vi "Text_help.vi"(6 "Onto":bool[](array[boolean]), 7 "Trigger Array":bool[](array[boolean]), 9 "Changed":bool, 10 "Bounds":T2[](array[typedef]), 11 "Refs cluster In":T1) -> (3 "Refs cluster Out":T1)   [LabVIEW 2015]
uses:
  <vilib>/Utility/miscctls.llb/LVRectTypeDef.ctl
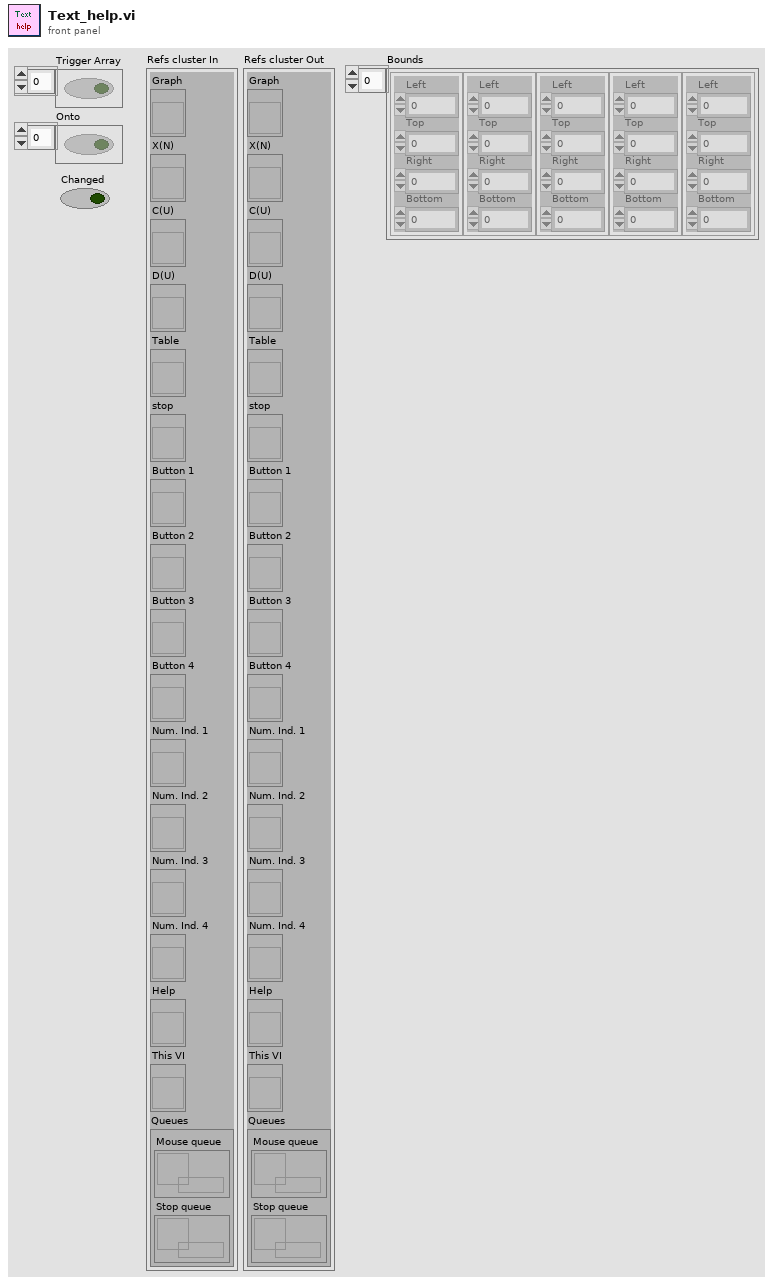
[diagram p1: front panel]
types:
  T1 = cluster{"Graph":refnum<vi>, "X(N)":refnum<vi>, "C(U)":refnum<vi>, "D(U)":refnum<vi>, "Table":refnum<vi>, "stop":refnum<vi>, "Button 1":refnum<vi>, "Button 2":refnum<vi>, "Button 3":refnum<vi>, "Button 4":refnum<vi>, "Num. Ind. 1":refnum<vi>, "Num. Ind. 2":refnum<vi>, "Num. Ind. 3":refnum<vi>, "Num. Ind. 4":refnum<vi>, "Help":refnum<vi>, "This VI":refnum<vi>, "Queues":cluster{"Mouse queue":refnum<queue>, "Stop queue":refnum<queue>}}
  T2 = typedef "LVRectTypeDef.ctl" = cluster{"Left":i16, "Top":i16, "Right":i16, "Bottom":i16}
  T3 = enum16{"top-left", "top-right", "bot-left", "bot-right"}
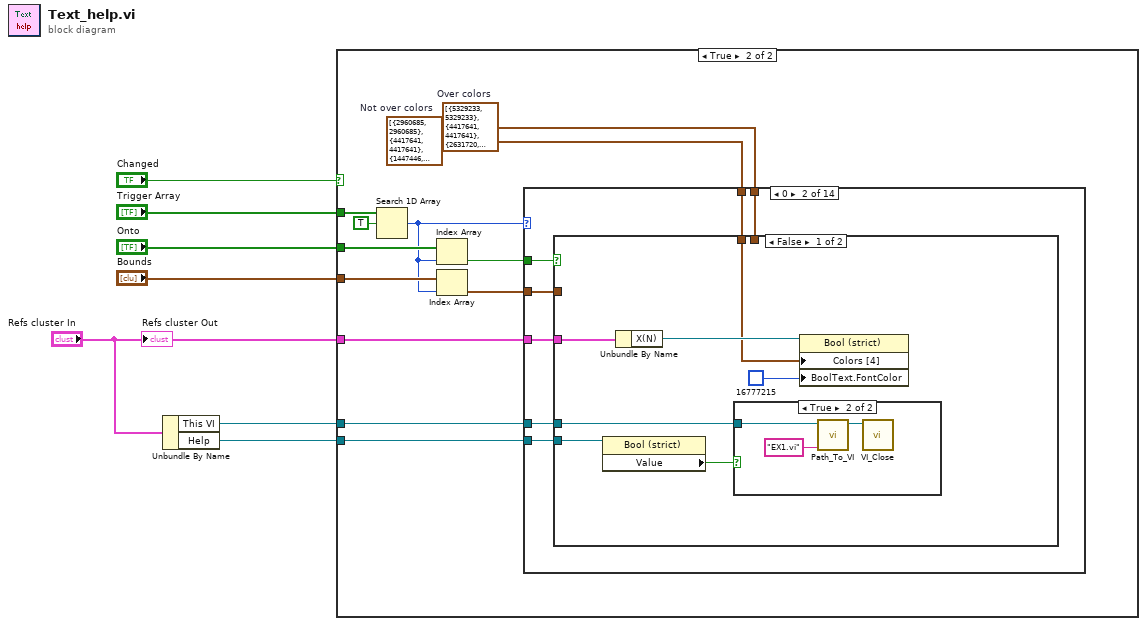
[diagram p0: block diagram]
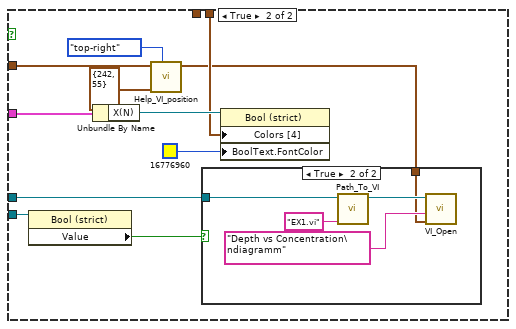
[diagram p5: hidden frame]
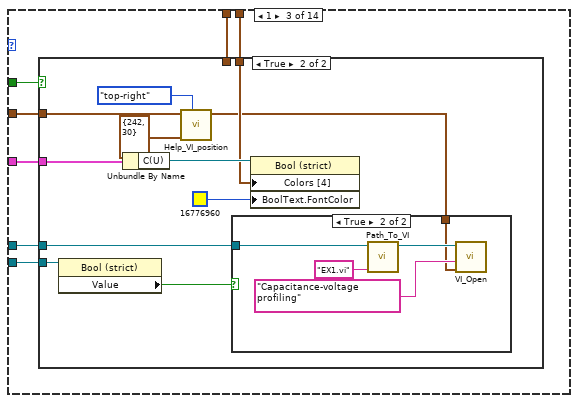
[diagram p7: hidden frame]
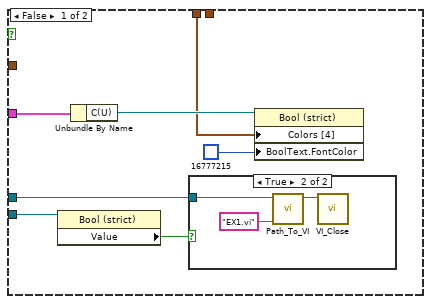
[diagram p8: hidden frame]
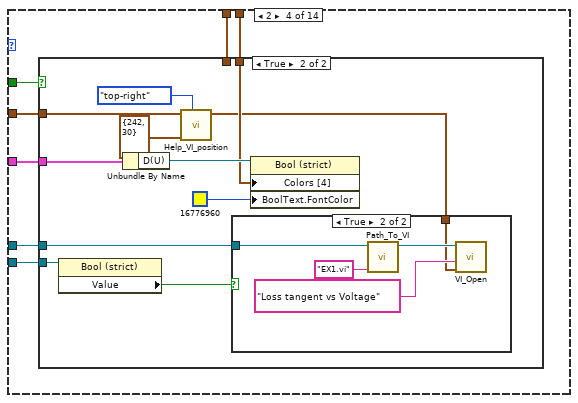
[diagram p11: hidden frame]
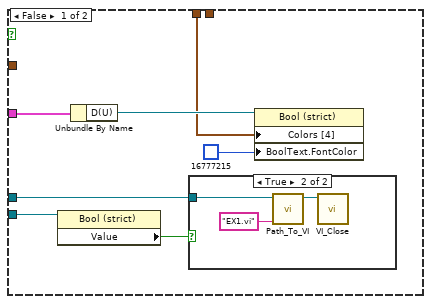
[diagram p12: hidden frame]
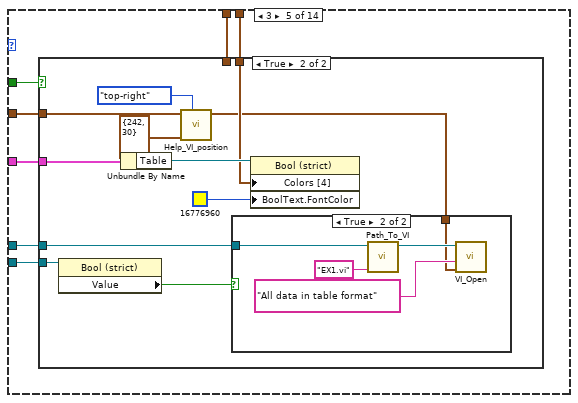
[diagram p15: hidden frame]
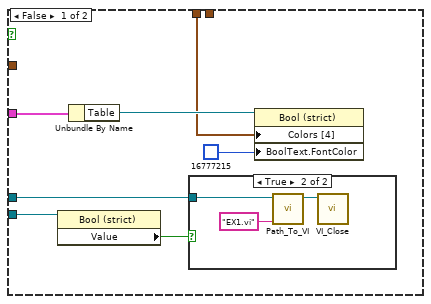
[diagram p16: hidden frame]
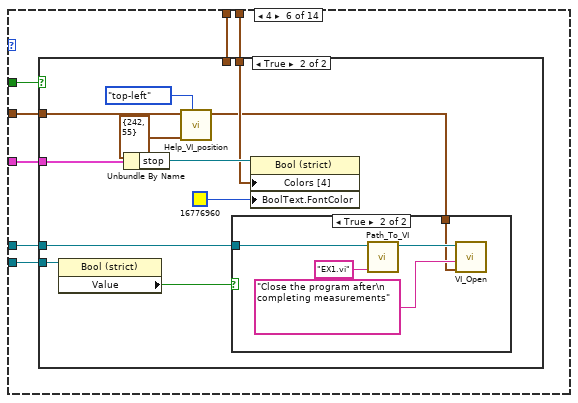
[diagram p19: hidden frame]
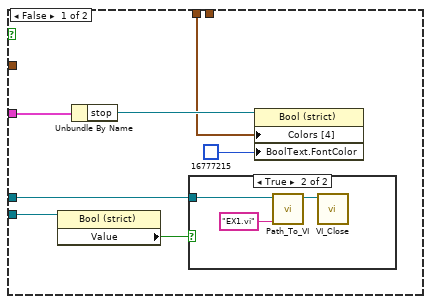
[diagram p20: hidden frame]
diagram:
  n1 = Unbundle By Name("Refs cluster In") -> ("This VI"=w2:refnum<vi>, "Help"=w1:refnum<vi>)
  n2 = case shown="True" "Changed" {
    tunnel: "Refs cluster In" -> [_ w15]
    tunnel: "Trigger Array" -> [_ w19]
    tunnel: "Onto" -> [_ w17]
    tunnel: "Bounds" -> [_ w14]
    tunnel: w2 -> [_ w9]
    tunnel: w1 -> [_ w8]
    frame False {
    }
    frame True {
      w10 = cluster{u32, u32}[] [{2960685, 2960685}, {4417641, 4417641}, {1447446, 1447446}, {2176052, 2176052}]  # Not over colors
      w11 = cluster{u32, u32}[] [{5329233, 5329233}, {4417641, 4417641}, {2631720, 2631720}, {2176052, 2176052}]  # Over colors
      n3 = Search 1D Array(1D array=w19, element=TRUE) -> (index of element=w13:i32)  [unwired: 1 in]
      n4 = Index Array(array=w17, index=w13) -> (element=w16:bool)
      n5 = Index Array(array=w14, index=w13) -> (element=w12:T2)
      n6 = case shown="0" w13 {
        tunnel: w16 -> [_ w25 w58 w91 w124 w157 w190 w223 w256 w289 w322 w355 w388 w421]
        tunnel: w15 -> [_ w26 w59 w92 w125 w158 w191 w224 w257 w290 w323 w356 w389 w422]
        tunnel: w12 -> [_ w24 w57 w90 w123 w156 w189 w222 w255 w288 w321 w354 w387 w420]
        tunnel: w11 -> [_ w22 w55 w88 w121 w154 w187 w220 w253 w286 w319 w352 w385 w418]
        tunnel: w10 -> [_ w21 w54 w87 w120 w153 w186 w219 w252 w285 w318 w351 w384 w417]
        tunnel: w9 -> [_ w23 w56 w89 w122 w155 w188 w221 w254 w287 w320 w353 w386 w419]
        tunnel: w8 -> [_ w20 w53 w86 w119 w152 w185 w218 w251 w284 w317 w350 w383 w416]
        frame -1, Default {
        }
        frame 0 {
          n7 = case shown="False" w25 {
            tunnel: w26 -> [w33 w47]
            tunnel: w24 -> [_ w40]
            tunnel: w23 -> [w29 w46]
            tunnel: w22 -> [_ w43]
            tunnel: w21 -> [w30 _]
            tunnel: w20 -> [w28 w38]
            frame False {
              n8 = property class="Bool (strict)"(reference=w28) -> ("Value"=w27:bool)  [unwired: 1 in, 2 out]
              n9 = Unbundle By Name(w33) -> ("X(N)"=w32:refnum<vi>)
              n10 = case shown="True" w27 {
                tunnel: w29 -> [_ w34]
                frame False {
                }
                frame True {
                  n11 = call "Path_To_VI.vi"("Vi name (with .vi)"="EX1.vi", "This Vi ref"=w34) -> ("Opening VI reference"=w36:refnum<vi>)  [unwired: 9 in]
                  n12 = call "VI_Close.vi"("VI_In"=w36) -> ()  [unwired: 10 in, 1 out]
                }
              }
              n13 = property on="Property Node" class="Bool (strict)"(reference=w32, "Colors [4]"=w30, "BoolText.FontColor"=u32 16777215) -> ()  [unwired: 1 in, 2 out]
            }
            frame True {
              n14 = property class="Bool (strict)"(reference=w38) -> ("Value"=w37:bool)  [unwired: 1 in, 2 out]
              n15 = Unbundle By Name(w47) -> ("X(N)"=w45:refnum<vi>)
              n16 = call "Help_VI_position.vi"("Enum"=T3."top-right", "Width-Height"=cluster{"width":i16, "height":i16} {"width"=242, "height"=55}, "Bounds button"=w40) -> ("Panel Bounds"=w39:T2)  [unwired: 8 in]
              n17 = case shown="True" w37 {
                tunnel: w46 -> [_ w49]
                tunnel: w39 -> [_ w48]
                frame False {
                }
                frame True {
                  n18 = call "Path_To_VI.vi"("Vi name (with .vi)"="EX1.vi", "This Vi ref"=w49) -> ("Opening VI reference"=w50:refnum<vi>)  [unwired: 9 in]
                  n19 = call "VI_Open.vi"("Panel Bounds"=w48, "Строка help"="Depth vs Concentration\ndiagramm", "Current VI In"=w50) -> ()  [unwired: 8 in, 1 out]
                }
              }
              n20 = property on="Property Node" class="Bool (strict)"(reference=w45, "Colors [4]"=w43, "BoolText.FontColor"=u32 16776960) -> ()  [unwired: 1 in, 2 out]
            }
          }
        }
        frame 1 {
          n21 = case shown="True" w58 {
            tunnel: w59 -> [w66 w80]
            tunnel: w57 -> [_ w73]
            tunnel: w56 -> [w62 w79]
            tunnel: w55 -> [_ w76]
            tunnel: w54 -> [w63 _]
            tunnel: w53 -> [w61 w71]
            frame False {
              n22 = property class="Bool (strict)"(reference=w61) -> ("Value"=w60:bool)  [unwired: 1 in, 2 out]
              n23 = Unbundle By Name(w66) -> ("C(U)"=w65:refnum<vi>)
              n24 = case shown="True" w60 {
                tunnel: w62 -> [_ w67]
                frame False {
                }
                frame True {
                  n25 = call "Path_To_VI.vi"("Vi name (with .vi)"="EX1.vi", "This Vi ref"=w67) -> ("Opening VI reference"=w69:refnum<vi>)  [unwired: 9 in]
                  n26 = call "VI_Close.vi"("VI_In"=w69) -> ()  [unwired: 10 in, 1 out]
                }
              }
              n27 = property on="Property Node" class="Bool (strict)"(reference=w65, "Colors [4]"=w63, "BoolText.FontColor"=u32 16777215) -> ()  [unwired: 1 in, 2 out]
            }
            frame True {
              n28 = property class="Bool (strict)"(reference=w71) -> ("Value"=w70:bool)  [unwired: 1 in, 2 out]
              n29 = Unbundle By Name(w80) -> ("C(U)"=w78:refnum<vi>)
              n30 = call "Help_VI_position.vi"("Enum"=T3."top-right", "Width-Height"=cluster{"width":i16, "height":i16} {"width"=242, "height"=30}, "Bounds button"=w73) -> ("Panel Bounds"=w72:T2)  [unwired: 8 in]
              n31 = case shown="True" w70 {
                tunnel: w79 -> [_ w82]
                tunnel: w72 -> [_ w81]
                frame False {
                }
                frame True {
                  n32 = call "Path_To_VI.vi"("Vi name (with .vi)"="EX1.vi", "This Vi ref"=w82) -> ("Opening VI reference"=w83:refnum<vi>)  [unwired: 9 in]
                  n33 = call "VI_Open.vi"("Panel Bounds"=w81, "Строка help"="Capacitance-voltage profiling", "Current VI In"=w83) -> ()  [unwired: 8 in, 1 out]
                }
              }
              n34 = property on="Property Node" class="Bool (strict)"(reference=w78, "Colors [4]"=w76, "BoolText.FontColor"=u32 16776960) -> ()  [unwired: 1 in, 2 out]
            }
          }
        }
        frame 2 {
          n35 = case shown="True" w91 {
            tunnel: w92 -> [w99 w113]
            tunnel: w90 -> [_ w106]
            tunnel: w89 -> [w95 w112]
            tunnel: w88 -> [_ w109]
            tunnel: w87 -> [w96 _]
            tunnel: w86 -> [w94 w104]
            frame False {
              n36 = property class="Bool (strict)"(reference=w94) -> ("Value"=w93:bool)  [unwired: 1 in, 2 out]
              n37 = Unbundle By Name(w99) -> ("D(U)"=w98:refnum<vi>)
              n38 = case shown="True" w93 {
                tunnel: w95 -> [_ w100]
                frame False {
                }
                frame True {
                  n39 = call "Path_To_VI.vi"("Vi name (with .vi)"="EX1.vi", "This Vi ref"=w100) -> ("Opening VI reference"=w102:refnum<vi>)  [unwired: 9 in]
                  n40 = call "VI_Close.vi"("VI_In"=w102) -> ()  [unwired: 10 in, 1 out]
                }
              }
              n41 = property on="Property Node" class="Bool (strict)"(reference=w98, "Colors [4]"=w96, "BoolText.FontColor"=u32 16777215) -> ()  [unwired: 1 in, 2 out]
            }
            frame True {
              n42 = property class="Bool (strict)"(reference=w104) -> ("Value"=w103:bool)  [unwired: 1 in, 2 out]
              n43 = Unbundle By Name(w113) -> ("D(U)"=w111:refnum<vi>)
              n44 = call "Help_VI_position.vi"("Enum"=T3."top-right", "Width-Height"=cluster{"width":i16, "height":i16} {"width"=242, "height"=30}, "Bounds button"=w106) -> ("Panel Bounds"=w105:T2)  [unwired: 8 in]
              n45 = case shown="True" w103 {
                tunnel: w112 -> [_ w115]
                tunnel: w105 -> [_ w114]
                frame False {
                }
                frame True {
                  n46 = call "Path_To_VI.vi"("Vi name (with .vi)"="EX1.vi", "This Vi ref"=w115) -> ("Opening VI reference"=w116:refnum<vi>)  [unwired: 9 in]
                  n47 = call "VI_Open.vi"("Panel Bounds"=w114, "Строка help"="Loss tangent vs Voltage", "Current VI In"=w116) -> ()  [unwired: 8 in, 1 out]
                }
              }
              n48 = property on="Property Node" class="Bool (strict)"(reference=w111, "Colors [4]"=w109, "BoolText.FontColor"=u32 16776960) -> ()  [unwired: 1 in, 2 out]
            }
          }
        }
        frame 3 {
          n49 = case shown="True" w124 {
            tunnel: w125 -> [w132 w146]
            tunnel: w123 -> [_ w139]
            tunnel: w122 -> [w128 w145]
            tunnel: w121 -> [_ w142]
            tunnel: w120 -> [w129 _]
            tunnel: w119 -> [w127 w137]
            frame False {
              n50 = property class="Bool (strict)"(reference=w127) -> ("Value"=w126:bool)  [unwired: 1 in, 2 out]
              n51 = Unbundle By Name(w132) -> ("Table"=w131:refnum<vi>)
              n52 = case shown="True" w126 {
                tunnel: w128 -> [_ w133]
                frame False {
                }
                frame True {
                  n53 = call "Path_To_VI.vi"("Vi name (with .vi)"="EX1.vi", "This Vi ref"=w133) -> ("Opening VI reference"=w135:refnum<vi>)  [unwired: 9 in]
                  n54 = call "VI_Close.vi"("VI_In"=w135) -> ()  [unwired: 10 in, 1 out]
                }
              }
              n55 = property on="Property Node" class="Bool (strict)"(reference=w131, "Colors [4]"=w129, "BoolText.FontColor"=u32 16777215) -> ()  [unwired: 1 in, 2 out]
            }
            frame True {
              n56 = property class="Bool (strict)"(reference=w137) -> ("Value"=w136:bool)  [unwired: 1 in, 2 out]
              n57 = Unbundle By Name(w146) -> ("Table"=w144:refnum<vi>)
              n58 = call "Help_VI_position.vi"("Enum"=T3."top-right", "Width-Height"=cluster{"width":i16, "height":i16} {"width"=242, "height"=30}, "Bounds button"=w139) -> ("Panel Bounds"=w138:T2)  [unwired: 8 in]
              n59 = case shown="True" w136 {
                tunnel: w145 -> [_ w148]
                tunnel: w138 -> [_ w147]
                frame False {
                }
                frame True {
                  n60 = call "Path_To_VI.vi"("Vi name (with .vi)"="EX1.vi", "This Vi ref"=w148) -> ("Opening VI reference"=w149:refnum<vi>)  [unwired: 9 in]
                  n61 = call "VI_Open.vi"("Panel Bounds"=w147, "Строка help"="All data in table format", "Current VI In"=w149) -> ()  [unwired: 8 in, 1 out]
                }
              }
              n62 = property on="Property Node" class="Bool (strict)"(reference=w144, "Colors [4]"=w142, "BoolText.FontColor"=u32 16776960) -> ()  [unwired: 1 in, 2 out]
            }
          }
        }
        frame 4 {
          n63 = case shown="True" w157 {
            tunnel: w158 -> [w165 w179]
            tunnel: w156 -> [_ w172]
            tunnel: w155 -> [w161 w178]
            tunnel: w154 -> [_ w175]
            tunnel: w153 -> [w162 _]
            tunnel: w152 -> [w160 w170]
            frame False {
              n64 = property class="Bool (strict)"(reference=w160) -> ("Value"=w159:bool)  [unwired: 1 in, 2 out]
              n65 = Unbundle By Name(w165) -> ("stop"=w164:refnum<vi>)
              n66 = case shown="True" w159 {
                tunnel: w161 -> [_ w166]
                frame False {
                }
                frame True {
                  n67 = call "Path_To_VI.vi"("Vi name (with .vi)"="EX1.vi", "This Vi ref"=w166) -> ("Opening VI reference"=w168:refnum<vi>)  [unwired: 9 in]
                  n68 = call "VI_Close.vi"("VI_In"=w168) -> ()  [unwired: 10 in, 1 out]
                }
              }
              n69 = property on="Property Node" class="Bool (strict)"(reference=w164, "Colors [4]"=w162, "BoolText.FontColor"=u32 16777215) -> ()  [unwired: 1 in, 2 out]
            }
            frame True {
              n70 = property class="Bool (strict)"(reference=w170) -> ("Value"=w169:bool)  [unwired: 1 in, 2 out]
              n71 = Unbundle By Name(w179) -> ("stop"=w177:refnum<vi>)
              n72 = call "Help_VI_position.vi"("Enum"=T3."top-left", "Width-Height"=cluster{"width":i16, "height":i16} {"width"=242, "height"=55}, "Bounds button"=w172) -> ("Panel Bounds"=w171:T2)  [unwired: 8 in]
              n73 = case shown="True" w169 {
                tunnel: w178 -> [_ w181]
                tunnel: w171 -> [_ w180]
                frame False {
                }
                frame True {
                  n74 = call "Path_To_VI.vi"("Vi name (with .vi)"="EX1.vi", "This Vi ref"=w181) -> ("Opening VI reference"=w182:refnum<vi>)  [unwired: 9 in]
                  n75 = call "VI_Open.vi"("Panel Bounds"=w180, "Строка help"="Close the program after\n completing measurements", "Current VI In"=w182) -> ()  [unwired: 8 in, 1 out]
                }
              }
              n76 = property on="Property Node" class="Bool (strict)"(reference=w177, "Colors [4]"=w175, "BoolText.FontColor"=u32 16776960) -> ()  [unwired: 1 in, 2 out]
            }
          }
        }
        frame 5 {
          n77 = case shown="True" w190 {
            tunnel: w191 -> [w198 w212]
            tunnel: w189 -> [_ w205]
            tunnel: w188 -> [w194 w211]
            tunnel: w187 -> [_ w208]
            tunnel: w186 -> [w195 _]
            tunnel: w185 -> [w193 w203]
            frame False {
              n78 = property class="Bool (strict)"(reference=w193) -> ("Value"=w192:bool)  [unwired: 1 in, 2 out]
              n79 = Unbundle By Name(w198) -> ("Button 1"=w197:refnum<vi>)
              n80 = case shown="True" w192 {
                tunnel: w194 -> [_ w199]
                frame False {
                }
                frame True {
                  n81 = call "Path_To_VI.vi"("Vi name (with .vi)"="EX1.vi", "This Vi ref"=w199) -> ("Opening VI reference"=w201:refnum<vi>)  [unwired: 9 in]
                  n82 = call "VI_Close.vi"("VI_In"=w201) -> ()  [unwired: 10 in, 1 out]
                }
              }
              n83 = property on="Property Node" class="Bool (strict)"(reference=w197, "Colors [4]"=w195, "BoolText.FontColor"=u32 16777215) -> ()  [unwired: 1 in, 2 out]
            }
            frame True {
              n84 = property class="Bool (strict)"(reference=w203) -> ("Value"=w202:bool)  [unwired: 1 in, 2 out]
              n85 = Unbundle By Name(w212) -> ("Button 1"=w210:refnum<vi>)
              n86 = call "Help_VI_position.vi"("Enum"=T3."bot-left", "Width-Height"=cluster{"width":i16, "height":i16} {"width"=242, "height"=30}, "Bounds button"=w205) -> ("Panel Bounds"=w204:T2)  [unwired: 8 in]
              n87 = case shown="True" w202 {
                tunnel: w211 -> [_ w214]
                tunnel: w204 -> [_ w213]
                frame False {
                }
                frame True {
                  n88 = call "Path_To_VI.vi"("Vi name (with .vi)"="EX1.vi", "This Vi ref"=w214) -> ("Opening VI reference"=w215:refnum<vi>)  [unwired: 9 in]
                  n89 = call "VI_Open.vi"("Panel Bounds"=w213, "Строка help"="Text for button #1", "Current VI In"=w215) -> ()  [unwired: 8 in, 1 out]
                }
              }
              n90 = property on="Property Node" class="Bool (strict)"(reference=w210, "Colors [4]"=w208, "BoolText.FontColor"=u32 16776960) -> ()  [unwired: 1 in, 2 out]
            }
          }
        }
        frame 6 {
          n91 = case shown="True" w223 {
            tunnel: w224 -> [w231 w245]
            tunnel: w222 -> [_ w238]
            tunnel: w221 -> [w227 w244]
            tunnel: w220 -> [_ w241]
            tunnel: w219 -> [w228 _]
            tunnel: w218 -> [w226 w236]
            frame False {
              n92 = property class="Bool (strict)"(reference=w226) -> ("Value"=w225:bool)  [unwired: 1 in, 2 out]
              n93 = Unbundle By Name(w231) -> ("Button 2"=w230:refnum<vi>)
              n94 = case shown="True" w225 {
                tunnel: w227 -> [_ w232]
                frame False {
                }
                frame True {
                  n95 = call "Path_To_VI.vi"("Vi name (with .vi)"="EX1.vi", "This Vi ref"=w232) -> ("Opening VI reference"=w234:refnum<vi>)  [unwired: 9 in]
                  n96 = call "VI_Close.vi"("VI_In"=w234) -> ()  [unwired: 10 in, 1 out]
                }
              }
              n97 = property on="Property Node" class="Bool (strict)"(reference=w230, "Colors [4]"=w228, "BoolText.FontColor"=u32 16777215) -> ()  [unwired: 1 in, 2 out]
            }
            frame True {
              n98 = property class="Bool (strict)"(reference=w236) -> ("Value"=w235:bool)  [unwired: 1 in, 2 out]
              n99 = Unbundle By Name(w245) -> ("Button 2"=w243:refnum<vi>)
              n100 = call "Help_VI_position.vi"("Enum"=T3."top-left", "Width-Height"=cluster{"width":i16, "height":i16} {"width"=242, "height"=30}, "Bounds button"=w238) -> ("Panel Bounds"=w237:T2)  [unwired: 8 in]
              n101 = case shown="True" w235 {
                tunnel: w244 -> [_ w247]
                tunnel: w237 -> [_ w246]
                frame False {
                }
                frame True {
                  n102 = call "Path_To_VI.vi"("Vi name (with .vi)"="EX1.vi", "This Vi ref"=w247) -> ("Opening VI reference"=w248:refnum<vi>)  [unwired: 9 in]
                  n103 = call "VI_Open.vi"("Panel Bounds"=w246, "Строка help"="Text for button #2", "Current VI In"=w248) -> ()  [unwired: 8 in, 1 out]
                }
              }
              n104 = property on="Property Node" class="Bool (strict)"(reference=w243, "Colors [4]"=w241, "BoolText.FontColor"=u32 16776960) -> ()  [unwired: 1 in, 2 out]
            }
          }
        }
        frame 7 {
          n105 = case shown="True" w256 {
            tunnel: w257 -> [w264 w278]
            tunnel: w255 -> [_ w271]
            tunnel: w254 -> [w260 w277]
            tunnel: w253 -> [_ w274]
            tunnel: w252 -> [w261 _]
            tunnel: w251 -> [w259 w269]
            frame False {
              n106 = property class="Bool (strict)"(reference=w259) -> ("Value"=w258:bool)  [unwired: 1 in, 2 out]
              n107 = Unbundle By Name(w264) -> ("Button 3"=w263:refnum<vi>)
              n108 = case shown="True" w258 {
                tunnel: w260 -> [_ w265]
                frame False {
                }
                frame True {
                  n109 = call "Path_To_VI.vi"("Vi name (with .vi)"="EX1.vi", "This Vi ref"=w265) -> ("Opening VI reference"=w267:refnum<vi>)  [unwired: 9 in]
                  n110 = call "VI_Close.vi"("VI_In"=w267) -> ()  [unwired: 10 in, 1 out]
                }
              }
              n111 = property on="Property Node" class="Bool (strict)"(reference=w263, "Colors [4]"=w261, "BoolText.FontColor"=u32 16777215) -> ()  [unwired: 1 in, 2 out]
            }
            frame True {
              n112 = property class="Bool (strict)"(reference=w269) -> ("Value"=w268:bool)  [unwired: 1 in, 2 out]
              n113 = Unbundle By Name(w278) -> ("Button 3"=w276:refnum<vi>)
              n114 = call "Help_VI_position.vi"("Enum"=T3."top-left", "Width-Height"=cluster{"width":i16, "height":i16} {"width"=242, "height"=30}, "Bounds button"=w271) -> ("Panel Bounds"=w270:T2)  [unwired: 8 in]
              n115 = case shown="True" w268 {
                tunnel: w277 -> [_ w280]
                tunnel: w270 -> [_ w279]
                frame False {
                }
                frame True {
                  n116 = call "Path_To_VI.vi"("Vi name (with .vi)"="EX1.vi", "This Vi ref"=w280) -> ("Opening VI reference"=w281:refnum<vi>)  [unwired: 9 in]
                  n117 = call "VI_Open.vi"("Panel Bounds"=w279, "Строка help"="Text for button #3", "Current VI In"=w281) -> ()  [unwired: 8 in, 1 out]
                }
              }
              n118 = property on="Property Node" class="Bool (strict)"(reference=w276, "Colors [4]"=w274, "BoolText.FontColor"=u32 16776960) -> ()  [unwired: 1 in, 2 out]
            }
          }
        }
        frame 8 {
          n119 = case shown="True" w289 {
            tunnel: w290 -> [w297 w311]
            tunnel: w288 -> [_ w304]
            tunnel: w287 -> [w293 w310]
            tunnel: w286 -> [_ w307]
            tunnel: w285 -> [w294 _]
            tunnel: w284 -> [w292 w302]
            frame False {
              n120 = property class="Bool (strict)"(reference=w292) -> ("Value"=w291:bool)  [unwired: 1 in, 2 out]
              n121 = Unbundle By Name(w297) -> ("Button 4"=w296:refnum<vi>)
              n122 = case shown="True" w291 {
                tunnel: w293 -> [_ w298]
                frame False {
                }
                frame True {
                  n123 = call "Path_To_VI.vi"("Vi name (with .vi)"="EX1.vi", "This Vi ref"=w298) -> ("Opening VI reference"=w300:refnum<vi>)  [unwired: 9 in]
                  n124 = call "VI_Close.vi"("VI_In"=w300) -> ()  [unwired: 10 in, 1 out]
                }
              }
              n125 = property on="Property Node" class="Bool (strict)"(reference=w296, "Colors [4]"=w294, "BoolText.FontColor"=u32 16777215) -> ()  [unwired: 1 in, 2 out]
            }
            frame True {
              n126 = property class="Bool (strict)"(reference=w302) -> ("Value"=w301:bool)  [unwired: 1 in, 2 out]
              n127 = Unbundle By Name(w311) -> ("Button 4"=w309:refnum<vi>)
              n128 = call "Help_VI_position.vi"("Enum"=T3."top-left", "Width-Height"=cluster{"width":i16, "height":i16} {"width"=242, "height"=30}, "Bounds button"=w304) -> ("Panel Bounds"=w303:T2)  [unwired: 8 in]
              n129 = case shown="True" w301 {
                tunnel: w310 -> [_ w313]
                tunnel: w303 -> [_ w312]
                frame False {
                }
                frame True {
                  n130 = call "Path_To_VI.vi"("Vi name (with .vi)"="EX1.vi", "This Vi ref"=w313) -> ("Opening VI reference"=w314:refnum<vi>)  [unwired: 9 in]
                  n131 = call "VI_Open.vi"("Panel Bounds"=w312, "Строка help"="Text for button #4", "Current VI In"=w314) -> ()  [unwired: 8 in, 1 out]
                }
              }
              n132 = property on="Property Node" class="Bool (strict)"(reference=w309, "Colors [4]"=w307, "BoolText.FontColor"=u32 16776960) -> ()  [unwired: 1 in, 2 out]
            }
          }
        }
        frame 9 {
          n133 = case shown="True" w322 {
            tunnel: w323 -> [w330 w344]
            tunnel: w321 -> [_ w340]
            tunnel: w320 -> [w329 w343]
            tunnel: w319 -> [_ _]
            tunnel: w318 -> [_ _]
            tunnel: w317 -> [w328 w338]
            frame False {
              n134 = Unbundle By Name(w330) -> ("Num. Ind. 1"=w324:refnum<vi>)
              n135 = property class="Bool (strict)"(reference=w328) -> ("Value"=w327:bool)  [unwired: 1 in, 2 out]
              n136 = property on="Property Node" class="DigNum (strict)"(reference=w324, "NumText.TextColors"=cluster{u32, u32} {16777215, 3815994} ("Cluster"), "Label.TextColor"=u32 16777215) -> ()  [unwired: 1 in, 2 out]
              n137 = case shown="True" w327 {
                tunnel: w329 -> [_ w331]
                frame False {
                }
                frame True {
                  n138 = call "Path_To_VI.vi"("Vi name (with .vi)"="EX1.vi", "This Vi ref"=w331) -> ("Opening VI reference"=w333:refnum<vi>)  [unwired: 9 in]
                  n139 = call "VI_Close.vi"("VI_In"=w333) -> ()  [unwired: 10 in, 1 out]
                }
              }
            }
            frame True {
              n140 = property class="Bool (strict)"(reference=w338) -> ("Value"=w337:bool)  [unwired: 1 in, 2 out]
              n141 = Unbundle By Name(w344) -> ("Num. Ind. 1"=w335:refnum<vi>)
              n142 = call "Help_VI_position.vi"("Enum"=T3."bot-left", "Width-Height"=cluster{"width":i16, "height":i16} {"width"=242, "height"=30}, "Bounds button"=w340) -> ("Panel Bounds"=w339:T2)  [unwired: 8 in]
              n143 = case shown="True" w337 {
                tunnel: w343 -> [_ w346]
                tunnel: w339 -> [_ w345]
                frame False {
                }
                frame True {
                  n144 = call "Path_To_VI.vi"("Vi name (with .vi)"="EX1.vi", "This Vi ref"=w346) -> ("Opening VI reference"=w347:refnum<vi>)  [unwired: 9 in]
                  n145 = call "VI_Open.vi"("Panel Bounds"=w345, "Строка help"="Text for Numeric Indicator #1", "Current VI In"=w347) -> ()  [unwired: 8 in, 1 out]
                }
              }
              n146 = property on="Property Node" class="DigNum (strict)"(reference=w335, "NumText.TextColors"=cluster{u32, u32} {16645629, 5263440}, "Label.TextColor"=u32 16776960) -> ()  [unwired: 1 in, 2 out]
            }
          }
        }
        frame 10 {
          n147 = case shown="True" w355 {
            tunnel: w356 -> [w363 w377]
            tunnel: w354 -> [_ w373]
            tunnel: w353 -> [w362 w376]
            tunnel: w352 -> [_ _]
            tunnel: w351 -> [_ _]
            tunnel: w350 -> [w361 w371]
            frame False {
              n148 = Unbundle By Name(w363) -> ("Num. Ind. 2"=w357:refnum<vi>)
              n149 = property class="Bool (strict)"(reference=w361) -> ("Value"=w360:bool)  [unwired: 1 in, 2 out]
              n150 = property on="Property Node" class="DigNum (strict)"(reference=w357, "NumText.TextColors"=cluster{u32, u32} {16777215, 3815994} ("Cluster"), "Label.TextColor"=u32 16777215) -> ()  [unwired: 1 in, 2 out]
              n151 = case shown="True" w360 {
                tunnel: w362 -> [_ w364]
                frame False {
                }
                frame True {
                  n152 = call "Path_To_VI.vi"("Vi name (with .vi)"="EX1.vi", "This Vi ref"=w364) -> ("Opening VI reference"=w366:refnum<vi>)  [unwired: 9 in]
                  n153 = call "VI_Close.vi"("VI_In"=w366) -> ()  [unwired: 10 in, 1 out]
                }
              }
            }
            frame True {
              n154 = property class="Bool (strict)"(reference=w371) -> ("Value"=w370:bool)  [unwired: 1 in, 2 out]
              n155 = Unbundle By Name(w377) -> ("Num. Ind. 2"=w368:refnum<vi>)
              n156 = call "Help_VI_position.vi"("Enum"=T3."bot-left", "Width-Height"=cluster{"width":i16, "height":i16} {"width"=242, "height"=30}, "Bounds button"=w373) -> ("Panel Bounds"=w372:T2)  [unwired: 8 in]
              n157 = case shown="True" w370 {
                tunnel: w376 -> [_ w379]
                tunnel: w372 -> [_ w378]
                frame False {
                }
                frame True {
                  n158 = call "Path_To_VI.vi"("Vi name (with .vi)"="EX1.vi", "This Vi ref"=w379) -> ("Opening VI reference"=w380:refnum<vi>)  [unwired: 9 in]
                  n159 = call "VI_Open.vi"("Panel Bounds"=w378, "Строка help"="Text for Numeric Indicator #2", "Current VI In"=w380) -> ()  [unwired: 8 in, 1 out]
                }
              }
              n160 = property on="Property Node" class="DigNum (strict)"(reference=w368, "NumText.TextColors"=cluster{u32, u32} {16645629, 5263440}, "Label.TextColor"=u32 16776960) -> ()  [unwired: 1 in, 2 out]
            }
          }
        }
        frame 11 {
          n161 = case shown="True" w388 {
            tunnel: w389 -> [w396 w410]
            tunnel: w387 -> [_ w406]
            tunnel: w386 -> [w395 w409]
            tunnel: w385 -> [_ _]
            tunnel: w384 -> [_ _]
            tunnel: w383 -> [w394 w404]
            frame False {
              n162 = Unbundle By Name(w396) -> ("Num. Ind. 3"=w390:refnum<vi>)
              n163 = property class="Bool (strict)"(reference=w394) -> ("Value"=w393:bool)  [unwired: 1 in, 2 out]
              n164 = property on="Property Node" class="DigNum (strict)"(reference=w390, "NumText.TextColors"=cluster{u32, u32} {16777215, 3815994} ("Cluster"), "Label.TextColor"=u32 16777215) -> ()  [unwired: 1 in, 2 out]
              n165 = case shown="True" w393 {
                tunnel: w395 -> [_ w397]
                frame False {
                }
                frame True {
                  n166 = call "Path_To_VI.vi"("Vi name (with .vi)"="EX1.vi", "This Vi ref"=w397) -> ("Opening VI reference"=w399:refnum<vi>)  [unwired: 9 in]
                  n167 = call "VI_Close.vi"("VI_In"=w399) -> ()  [unwired: 10 in, 1 out]
                }
              }
            }
            frame True {
              n168 = property class="Bool (strict)"(reference=w404) -> ("Value"=w403:bool)  [unwired: 1 in, 2 out]
              n169 = Unbundle By Name(w410) -> ("Num. Ind. 3"=w401:refnum<vi>)
              n170 = call "Help_VI_position.vi"("Enum"=T3."top-left", "Width-Height"=cluster{"width":i16, "height":i16} {"width"=242, "height"=30}, "Bounds button"=w406) -> ("Panel Bounds"=w405:T2)  [unwired: 8 in]
              n171 = case shown="True" w403 {
                tunnel: w409 -> [_ w412]
                tunnel: w405 -> [_ w411]
                frame False {
                }
                frame True {
                  n172 = call "Path_To_VI.vi"("Vi name (with .vi)"="EX1.vi", "This Vi ref"=w412) -> ("Opening VI reference"=w413:refnum<vi>)  [unwired: 9 in]
                  n173 = call "VI_Open.vi"("Panel Bounds"=w411, "Строка help"="Text for Numeric Indicator #3", "Current VI In"=w413) -> ()  [unwired: 8 in, 1 out]
                }
              }
              n174 = property on="Property Node" class="DigNum (strict)"(reference=w401, "NumText.TextColors"=cluster{u32, u32} {16645629, 5263440}, "Label.TextColor"=u32 16776960) -> ()  [unwired: 1 in, 2 out]
            }
          }
        }
        frame 12 {
          n175 = case shown="True" w421 {
            tunnel: w422 -> [w429 w443]
            tunnel: w420 -> [_ w439]
            tunnel: w419 -> [w428 w442]
            tunnel: w418 -> [_ _]
            tunnel: w417 -> [_ _]
            tunnel: w416 -> [w427 w437]
            frame False {
              n176 = Unbundle By Name(w429) -> ("Num. Ind. 4"=w423:refnum<vi>)
              n177 = property class="Bool (strict)"(reference=w427) -> ("Value"=w426:bool)  [unwired: 1 in, 2 out]
              n178 = property on="Property Node" class="DigNum (strict)"(reference=w423, "NumText.TextColors"=cluster{u32, u32} {16777215, 3815994} ("Cluster"), "Label.TextColor"=u32 16777215) -> ()  [unwired: 1 in, 2 out]
              n179 = case shown="True" w426 {
                tunnel: w428 -> [_ w430]
                frame False {
                }
                frame True {
                  n180 = call "Path_To_VI.vi"("Vi name (with .vi)"="EX1.vi", "This Vi ref"=w430) -> ("Opening VI reference"=w432:refnum<vi>)  [unwired: 9 in]
                  n181 = call "VI_Close.vi"("VI_In"=w432) -> ()  [unwired: 10 in, 1 out]
                }
              }
            }
            frame True {
              n182 = property class="Bool (strict)"(reference=w437) -> ("Value"=w436:bool)  [unwired: 1 in, 2 out]
              n183 = Unbundle By Name(w443) -> ("Num. Ind. 4"=w434:refnum<vi>)
              n184 = call "Help_VI_position.vi"("Enum"=T3."top-left", "Width-Height"=cluster{"width":i16, "height":i16} {"width"=242, "height"=30}, "Bounds button"=w439) -> ("Panel Bounds"=w438:T2)  [unwired: 8 in]
              n185 = case shown="True" w436 {
                tunnel: w442 -> [_ w445]
                tunnel: w438 -> [_ w444]
                frame False {
                }
                frame True {
                  n186 = call "Path_To_VI.vi"("Vi name (with .vi)"="EX1.vi", "This Vi ref"=w445) -> ("Opening VI reference"=w446:refnum<vi>)  [unwired: 9 in]
                  n187 = call "VI_Open.vi"("Panel Bounds"=w444, "Строка help"="Text for Numeric Indicator #4", "Current VI In"=w446) -> ()  [unwired: 8 in, 1 out]
                }
              }
              n188 = property on="Property Node" class="DigNum (strict)"(reference=w434, "NumText.TextColors"=cluster{u32, u32} {16645629, 5263440}, "Label.TextColor"=u32 16776960) -> ()  [unwired: 1 in, 2 out]
            }
          }
        }
      }
    }
  }
  "Refs cluster Out" <- "Refs cluster In"
